vi "Build_Asylum_SetOutWavePair.vi"(6 "interpolation":i32, 7 "whichBank":i32, 8 "error in (no error)":errorcluster, 9 "Wave B":cluster{"channelStringB":string, "waveB":string}, 10 "Wave A":cluster{"channelStringA":string, "waveA":string}, 11 "eventString":string) -> (0 "error out":errorcluster, 3 "Command":string)   [LabVIEW 2019]
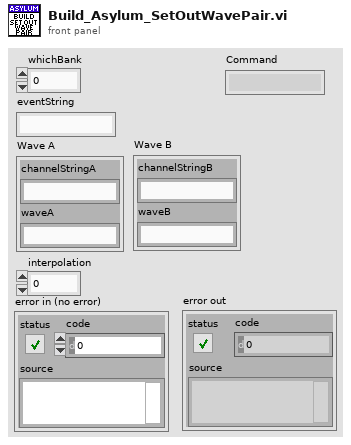
[diagram p1: front panel]
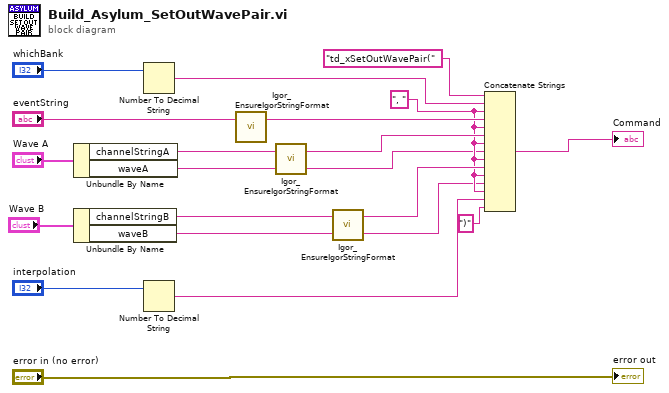
[diagram p0: block diagram]
diagram:
  w4 = ", " ("string")
  n1 = Unbundle By Name("Wave A") -> ("channelStringA"=w15:string, "waveA"=w1:string)
  n2 = Unbundle By Name("Wave B") -> ("channelStringB"=w6:string, "waveB"=w2:string)
  n3 = Number To Decimal String(number="whichBank") -> (decimal integer string=w13:string)  [unwired: 1 in]
  n4 = Number To Decimal String(number="interpolation") -> (decimal integer string=w10:string)  [unwired: 1 in]
  n5 = call "Igor_EnsureIgorStringFormat.vi"("Value"="eventString") -> ("Value"=w12:string)  [unwired: 2 in]
  n6 = call "Igor_EnsureIgorStringFormat.vi"("Value"=w15) -> ("Value"=w11:string)  [unwired: 2 in]
  n7 = call "Igor_EnsureIgorStringFormat.vi"("Value"=w6) -> ("Value"=w5:string)  [unwired: 2 in]
  n8 = Concatenate Strings("td_xSetOutWavePair(" ("string"), w13, w4, w12, w4, w11, w4, w1, w4, w5, w4, w2, w4, w10, ")" ("string")) -> (→"Command":string)
  "error out" <- "error in (no error)"
